vi "Test for Queue.vi"   [LabVIEW 2016, in "System.lvlib"]
uses:
  System.lvlib
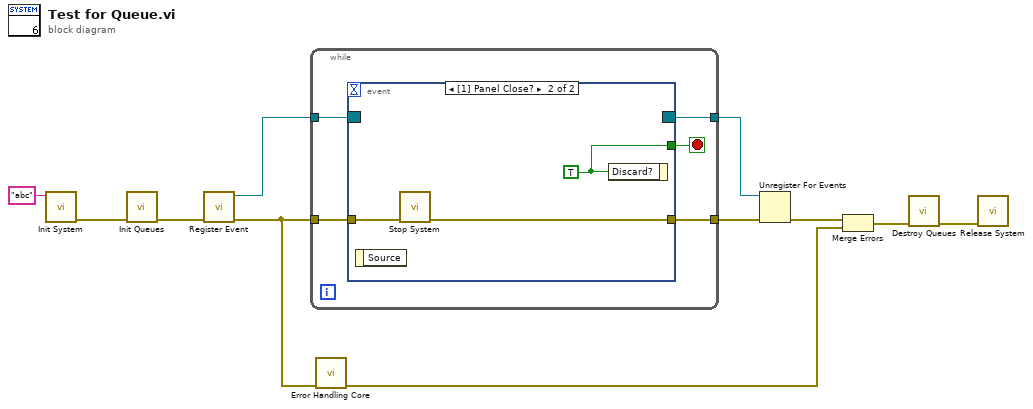
[diagram p0: block diagram]
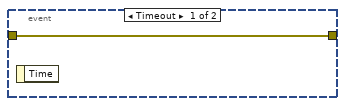
[diagram p2: hidden frame]
diagram:
  n1 = call "Init System.vi"("Application Name"="abc") -> ("error out"=w11:errorcluster)  [unwired: 10 in]
  n2 = call "Init Queues.vi"("error in (no error)"=w11) -> ("error out"=w10:errorcluster)  [unwired: 10 in]
  n3 = call "Register Event.vi"("error in (no error)"=w10) -> ("error out"=w8:errorcluster, "Event Registration Refnum"=w9:refnum<event-registration>)  [unwired: 9 in]
  n4 = while {
    tunnel: w8 -> [w16]
    tunnel: w9 -> [w15]
    tunnel: [w14] -> w5
    tunnel: [w12] -> w6
    stop <- w13 stop-if-true
    n5 = event shown="[1] Panel Close?" {
      selector: w15 -> [_ _]
      dyn-events: [_ _] -> w14
      timeout: _ -> [_ _]
      tunnel: w16 -> [w17 w19]
      tunnel: [_ w20] -> w13
      tunnel: [w17 w18] -> w12
      event Timeout {
        n6 = event-data() -> ()  [unwired: 1 in, 1 out]
      }
      event Panel Close? {
        w20 = TRUE
        n7 = event-data() -> ()  [unwired: 1 in, 1 out]
        n8 = call "Stop System.vi"("error in (no error)"=w19) -> ("error out"=w18:errorcluster)  [unwired: 10 in]
        n9 = event-data("Discard?"=w20) -> ()  [unwired: 1 in, 1 out]
      }
    }
  }
  n10 = call "Error Handling Core.vi"("error in (no error)"=w8) -> ("error out"=w3:errorcluster)  [unwired: 10 in]
  n11 = Unregister For Events(event registration refnum=w5, error in=w6) -> (error out=w4:errorcluster)
  n12 = Merge Errors(w4, w3) -> (w2:errorcluster)
  n13 = call "Destroy Queues.vi"("error in (no error)"=w2) -> ("error out"=w1:errorcluster)  [unwired: 10 in]
  n14 = call "Release System.vi"("error in (no error)"=w1) -> ()  [unwired: 10 in, 1 out]
